vi "IP Address List.vi"(6 "ignore Gateway IP?":bool=TRUE, 8 "error in (no error)":errorcluster) -> (0 "error out":errorcluster, 3 "Array":string[](array[string])=["192.168.5.5"])   [LabVIEW 2017]
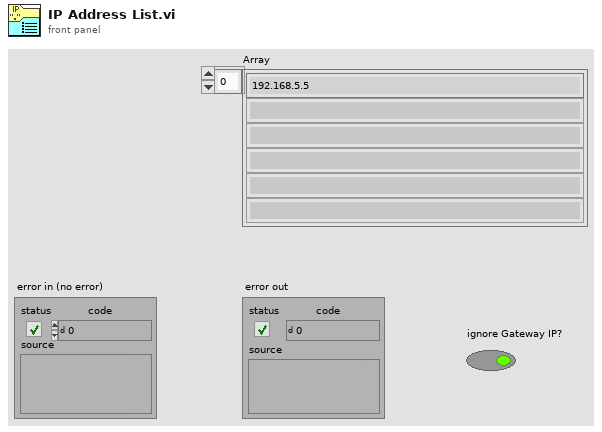
[diagram p1: front panel]
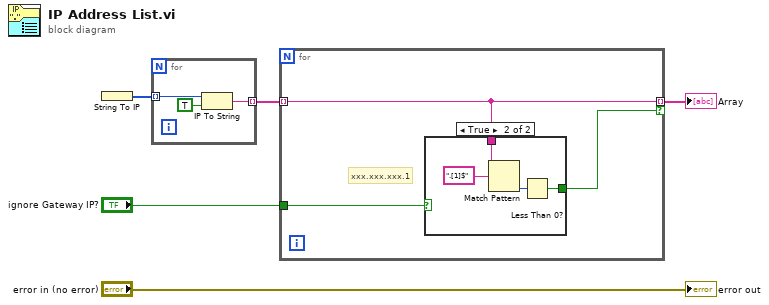
[diagram p0: block diagram]
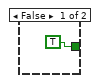
[diagram p2: hidden frame]
diagram:
  n1 = String To IP() -> (0:w1:u32[])  [unwired: 1 in]
  n2 = for {
    tunnel: w1 -> [w8] mode=indexing
    tunnel: [w6] -> w4 mode=indexing
    n3 = IP To String(1:TRUE ("dot notation? (F)"), 2:w8) -> (0:w6:string)
  }
  n4 = for {
    tunnel: w4 -> [w9] mode=indexing
    tunnel: [w9] -> w5 mode=indexing if=w10
    tunnel: "ignore Gateway IP?" -> [w11]
    # "xxx.xxx.xxx.1"
    n5 = case shown="True" w11 {
      tunnel: w9 -> [_ w15]
      tunnel: [TRUE w13] -> w10
      frame False {
      }
      frame True {
        n6 = Match Pattern(string=w15, regular expression=".[1]$") -> (offset past match=w14:i32)  [unwired: 1 in, 3 out]
        n7 = Less Than 0?(x=w14) -> (x < 0?=w13:bool)
      }
    }
  }
  "Array" <- w5
  "error out" <- "error in (no error)"
